vi "Pulse - Build Trigger.vi"(6 "Enabled":bool, 7 "Trigger Settings":T1, 8 "error in (no error)":errorcluster, 9 "Single Command In":string, 10 "Channel (1)":u32=1, 11 "3300 in":refnum<class "3300.lvclass">) -> (0 "error out":errorcluster, 1 "Single Command Out":string, 3 "3300 out":refnum<class "3300.lvclass">)   [LabVIEW 2019, in "3300.lvlib" / "3300.lvclass"]
uses:
  Library/3300.lvclass
  builds/Instruments/Electronic Load.lvlibp/Custom Controls/Trigger Settings.ctl
  builds/Instruments/Electronic Load.lvlibp/Custom Controls/E-Load Mode.ctl
  builds/Instruments/Electronic Load.lvlibp/Library/Electronic Load.lvclass
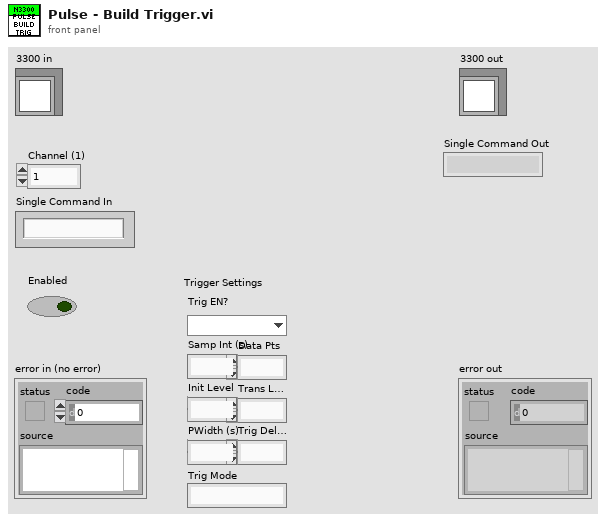
[diagram p1: front panel]
types:
  T1 = typedef "Electronic Load.lvlibp/Electronic Load.lvclass/Trigger Settings.ctl" = cluster{"Mode":T2, "Initial":dbl, "Transient":dbl, "Interval":dbl, "Width":dbl, "Delay":dbl, "Data Pts":i32, "Slew Rate":dbl}
  T2 = typedef "Electronic Load.lvlibp/Electronic Load.lvclass/E-Load Mode.ctl" = enum16{"Current", "Resistance", "Voltage"}
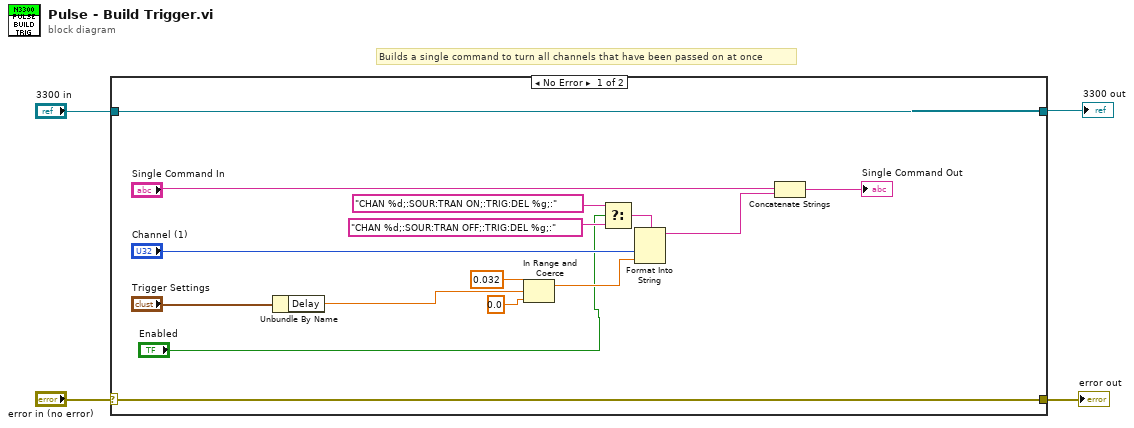
[diagram p0: block diagram]
diagram:
  # "Builds a single command to turn all channels that have been passed on at once"
  n1 = case shown="No Error" "error in (no error)" {
    selector: "error in (no error)" -> [w18 w21]
    tunnel: [w18 w21] -> w3
    tunnel: [w19 w20] -> w1
    tunnel: "3300 in" -> [w19 w20]
    frame No Error {
      n2 = Unbundle By Name("Trigger Settings") -> ("Delay"=w13:dbl)
      n3 = In Range and Coerce(upper limit=0.032, x=w13, lower limit=0.0) -> (coerced(x)=w14:dbl)  [unwired: 1 out]
      n4 = Select(t="CHAN %d;:SOUR:TRAN ON;:TRIG:DEL %g;:" ("format string"), s="Enabled", f="CHAN %d;:SOUR:TRAN OFF;:TRIG:DEL %g;:" ("format string")) -> (s? t:f=w10:string)
      n5 = Format Into String(format string=w10, "Channel (1)", w14) -> (resulting string=w17:string)  [unwired: 2 in, 1 out]
      n6 = Concatenate Strings("Single Command In", w17) -> (→"Single Command Out":string)
    }
    frame Error {
    }
  }
  "error out" <- w3
  "3300 out" <- w1
